vi "SimuFichEnCroissance.vi"() -> ()   [LabVIEW 2017]
panel:
  out "sortie d'erreur":errorcluster
  in  "chemin du fichier (utiliser une boîte de dialogue)":path
  in  "STOP":bool
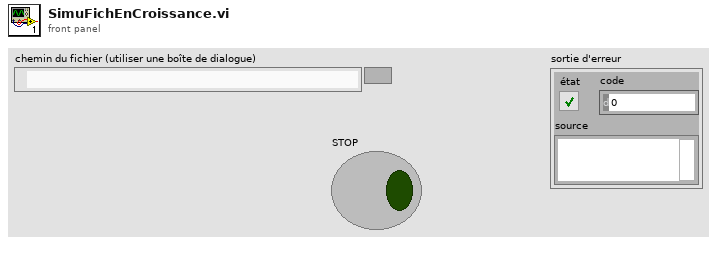
[diagram p1: front panel]
types:
  T1 = enum16{"open", "replace", "create", "open or create", "replace or create", "replace or create with confirmation"}
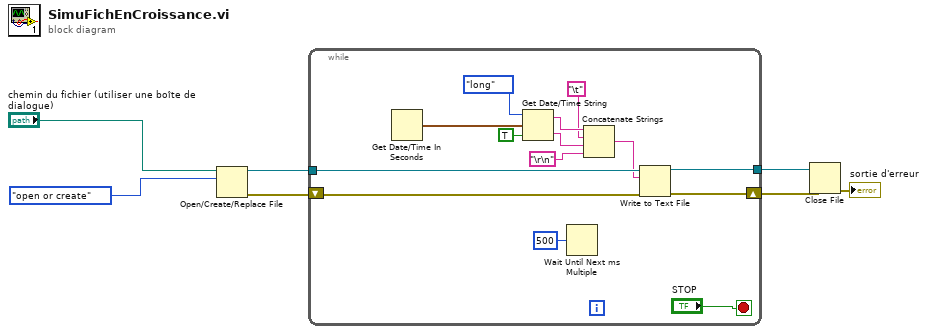
[diagram p0: block diagram]
diagram:
  n1 = Open/Create/Replace File(file path (use dialog)="chemin du fichier (utiliser une boîte de dialogue)", operation (0:open)=T1."open or create" ("opération (0 : open)")) -> (refnum out=w5:refnum<file>, error out=w7:errorcluster)  [unwired: 4 in, 1 out]
  n2 = while {
    shift-right: [w18] -> w6
    shift-left: w7 -> [w19]
    tunnel: w5 -> [w17]
    tunnel: [w16] -> w4
    stop <- "STOP" stop-if-true
    n3 = Get Date/Time In Seconds() -> (seconds since 1Jan1904=w12:timestamp)
    n4 = Get Date/Time String(date format (0)=enum16{"short", "long", "abbreviated"}."long" ("format de date (0)"), seconds (now)=w12, want seconds? (F)=TRUE ("secondes ? (F)")) -> (date string=w15:string, time string=w9:string)
    n5 = Wait Until Next ms Multiple(millisecond multiple=u32 500 ("n millisecondes")) -> ()  [unwired: 1 out]
    n6 = Concatenate Strings(w15, "\t", w9, "\r\n") -> (w14:string)
    n7 = Write to Text File(file (use dialog)=w17, text=w14, error in=w19) -> (refnum out=w16:refnum<file>, error out=w18:errorcluster)  [unwired: 1 in, 1 out]
  }
  n8 = Close File(refnum=w4, error in=w6) -> (error out=→"sortie d'erreur":errorcluster)  [unwired: 1 out]
